vi "tcs shm log Event Error Code LV.vi"(8 "error in (no error)":errorcluster, 11 "logevent_ErrorCode_Ctl":cluster{"errorCode":i32, "priority":i32}) -> (0 "error out":errorcluster, 2 "function return":i32, 3 "logevent_ErrorCode_Ctl out":cluster{"errorCode":i32, "priority":i32})   [LabVIEW 2016, in "SALLV_tcs.lvlib"]
doc: "int tcs_shm_logEvent_ErrorCodeLV(tcs_logevent_ErrorCodeLV *logevent_ErrorCode_Ctl );"
uses:
  SALLV_tcs.lvlib
  SALLV_tcs.so
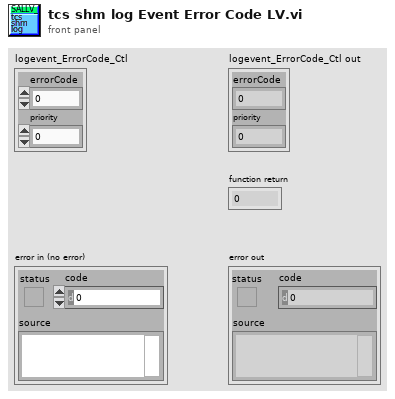
[diagram p1: front panel]
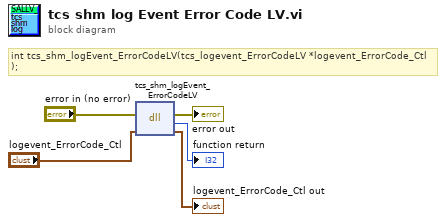
[diagram p0: block diagram]
diagram:
  # "int tcs_shm_logEvent_ErrorCodeLV(tcs_logevent_ErrorCodeLV *logevent_ErrorCode_Ctl );"
  n1 = dll-call lib="home/plotz/SALLV_tcs/SALLV_tcs.*" fn="tcs_shm_logEvent_ErrorCodeLV"(error in="error in (no error)", "logevent_ErrorCode_Ctl"="logevent_ErrorCode_Ctl") -> (error out=→"error out":errorcluster, →"function return":i32, "logevent_ErrorCode_Ctl"=→"logevent_ErrorCode_Ctl out":cluster{"errorCode":i32, "priority":i32})  [unwired: 2 in, 1 out]
